vi "Audio_Transformation_Setted_Frequency_v008.vi"() -> ()   [LabVIEW 2019]
uses:
  <vilib>/sound2/lvsound2.llb/Sound Data Format.ctl
  <vilib>/sound2/lvsound2.llb/Sound Input Read (DBL).vi
  <vilib>/addons/Time Frequency Analysis/Transform.llb/TFA Online Gabor Transform (Real).vi
  <vilib>/addons/_Advanced Signal Processing/NI_AdvSigProcTFA.lvlib
panel:
  out "u(t)":T1(graph)
  out "V(t)":T1(graph)
  out "Noise Speech":dbl[](graph)
  in  "Address selector":i32[](array[numeric])
  in  "Neuron Type":T2(ring)=enum."Phasic Spiking (PS)"
  out "max index(es)":i32
  out "max value":dbl
  out "Waveform Graph":dbl[](graph)
  out "Magnitude of Gabor Coefficients":dbl[][](graph)
  in  "Stop":bool
  # "Step two : Graph of the amplitude of the Gabor coefficient of the different bins"
  # "Step three : Spike Response of the neurons"
  # "Step one: Sound recorded from the computer"
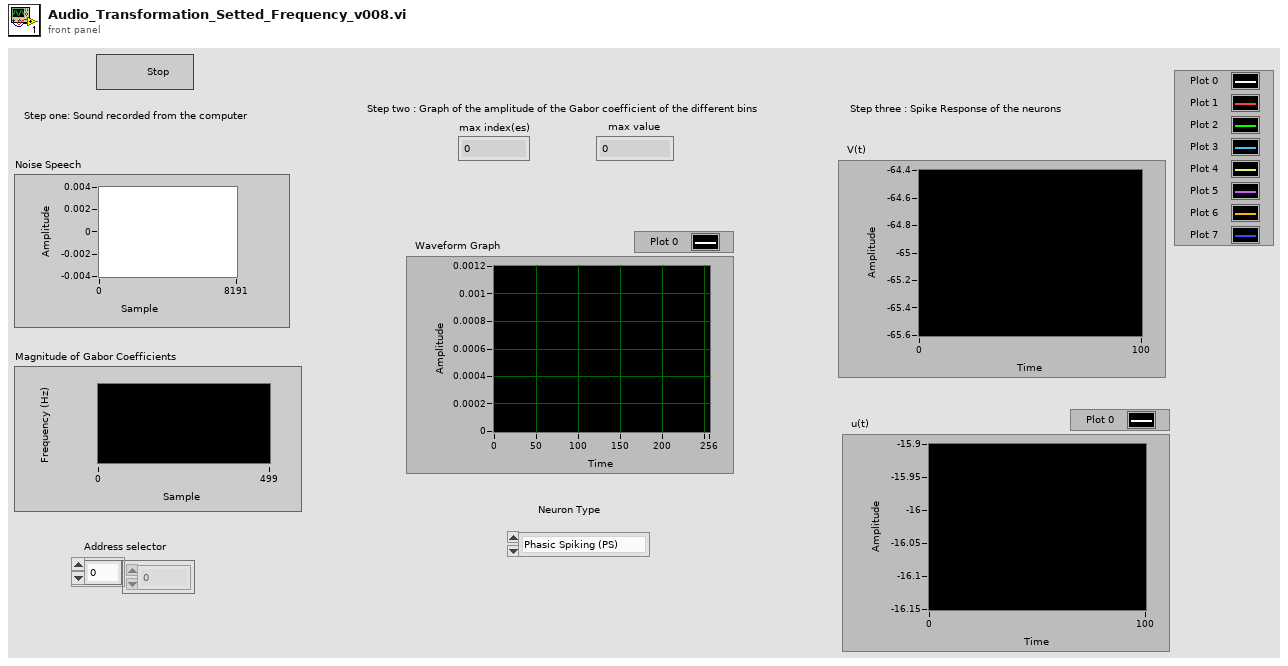
[diagram p1: front panel]
types:
  T1 = cluster{"[0]":dbl, "[1]":dbl, "[2]":dbl, "[3]":dbl, "[4]":dbl, "[5]":dbl, "[6]":dbl, "[7]":dbl}
  T2 = enum16{"Regular Spiking (RS)", "Intrinsically Bursting (IB)", "Chattering (CH)", "Fast Spiking (FS)", "Thalamo-Cortical 1 (TC1)", "Thalamo-Cortical 2 (TC2)", "Resonator (RZ)", "Low-Threshold Spiking (LTS)", "Phasic Spiking (PS)"}
  T3 = typedef "Sound Data Format.ctl" = cluster{"sample rate (S/s)":dbl, "number of channels":i32, "bits per sample":i32}
  T4 = cluster{"analysis window":dbl[], "dM (time steps)":i32, "N (frequency bins)":i32}
  T5 = typedef "Sound Input Task ID.ctl" = u32
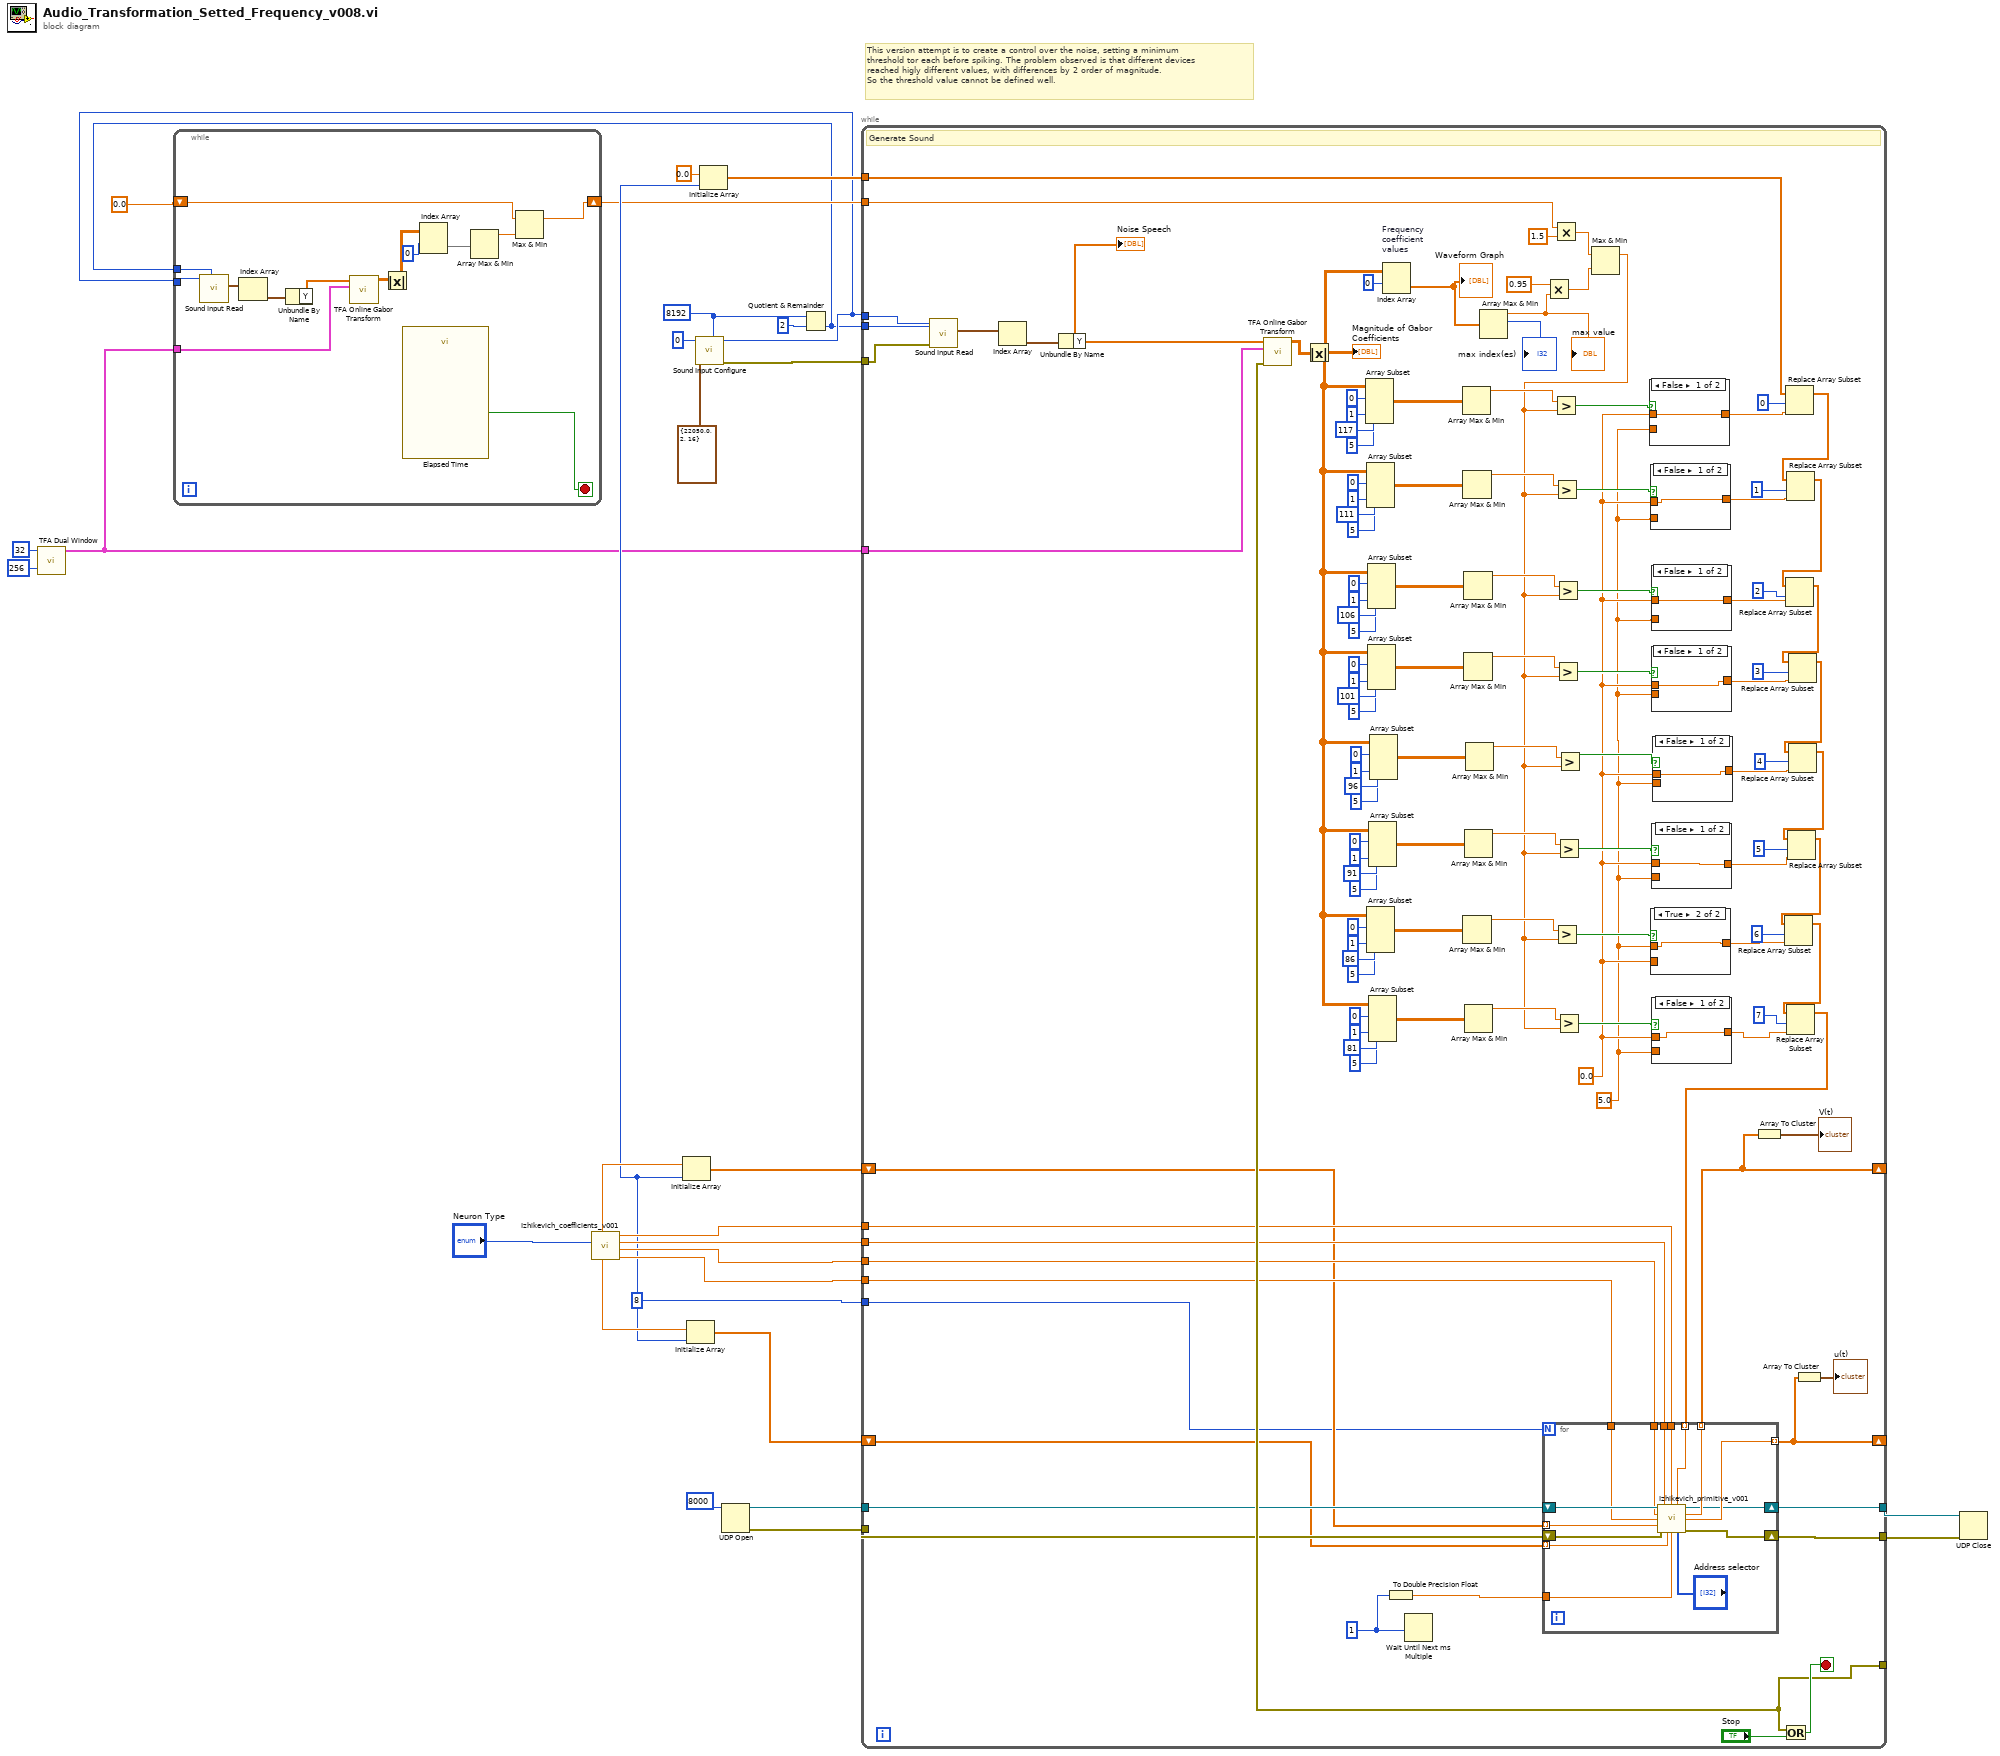
[diagram p0: block diagram]
diagram:
  w8 = 8
  w15 = 8192 ("number of samples/ch")
  # "This version attempt is to create a control over the noise, setting a minimum\nthreshold tor each before spiking. The problem observed is that different devices\nreached higly different values, with differences by 2 order of magnitude.\nSo the threshold value cannot be defined well."
  n1 = call <vilib>:"TFA Dual Window.vi"("N (frequency bins)"=256, "dM (time steps)"=32) -> ("analysis info"=w5:T4)  [unwired: 7 in, 2 out]
  n2 = call "Izhikevich_coefficients_v001.vi"("Neuron Type"="Neuron Type") -> ("d"=w23:dbl, "c"=w24:dbl, "b"=w25:dbl, "a"=w26:dbl, "u0"=w10:dbl, "v0"=w12:dbl)  [unwired: 3 in]
  n3 = Initialize Array(w12, w8) -> (w11:dbl[])
  n4 = Initialize Array(w10, w8) -> (w9:dbl[])
  n5 = call <vilib>:"Sound Input Configure.vi"("number of samples/ch"=w15, "sound format"=T3 {"sample rate (S/s)"=22050.0, "number of channels"=2, "bits per sample"=16}, "device ID"=u32 0) -> ("error out"=w13:errorcluster, "task ID"=w2:T5)  [unwired: 7 in]
  n6 = Initialize Array(0.0 ("element"), w8) -> (w6:dbl[])
  n7 = UDP Open(11:u16 8000 ("port")) -> (port=w21:refnum<k16>, 0:w20:errorcluster)  [unwired: 4 in, 1 out]
  n8 = Quotient & Remainder(x=w15, y=2) -> (floor(x/y)=w1:i32)  [unwired: 1 out]
  n9 = while {
    tunnel: w5 -> [w41]
    shift-right: [w33] -> w3
    shift-left: 0.0 -> [w34]
    tunnel: w2 -> [w31]
    tunnel: w1 -> [w30]
    stop <- w32 stop-if-true
    n10 = call-poly <vilib>:"Sound Input Read.vi"("number of samples/ch"=w30, "task ID"=w31) -> ("data"=w42:waveform(dbl)[])  [unwired: 7 in, 2 out]
    n11 = Index Array(array=w42) -> (element=w43:waveform(dbl))  [unwired: 1 in]
    n12 = Unbundle By Name(w43) -> ("Y"=w40:dbl[])
    n13 = call-poly <vilib>:"TFA Online Gabor Transform.vi"("transform info"=w41, "signal"=w40) -> ("Gabor coef"=w39:cdb[][])  [unwired: 7 in, 2 out]
    n14 = Absolute Value(x=w39) -> (abs(x)=w37:dbl[][])
    n15 = call "Elapsed Time"() -> ("Time has Elapsed"=w32:bool)  [unwired: 12 in, 7 out]
    n16 = Index Array(array=w37, index (row)=0) -> (element=w36:dbl[])  [unwired: 1 in]
    n17 = Array Max & Min(array=w36) -> (max value=w35:dbl)  [unwired: 3 out]
    n18 = Max & Min(x=w34, y=w35) -> (max(x,y)=w33:dbl)  [unwired: 1 out]
  }
  n19 = while {
    tunnel: [w158] -> _
    tunnel: w5 -> [w163]
    shift-right: [w57] -> _
    shift-left: w11 -> [w147]
    shift-right: [w55] -> _
    shift-left: w9 -> [w146]
    tunnel: w26 -> [w157]
    tunnel: w25 -> [w156]
    tunnel: w24 -> [w154]
    tunnel: w23 -> [w153]
    tunnel: w21 -> [w155]
    tunnel: w20 -> [w152]
    tunnel: [w149] -> w19
    tunnel: [w148] -> w18
    tunnel: w2 -> [w144]
    tunnel: w13 -> [w143]
    tunnel: w1 -> [w145]
    tunnel: w8 -> [w139]
    tunnel: w6 -> [w111]
    tunnel: w3 -> [w51]
    stop <- w164 stop-if-true
    w45 = 5.0
    w46 = 0.0
    w151 = u32 1 ("millisecond multiple")
    # "Generate Sound"
    n20 = call-poly <vilib>:"Sound Input Read.vi"("number of samples/ch"=w145, "error in (no error)"=w143, "task ID"=w144) -> ("data"=w141:waveform(dbl)[])  [unwired: 6 in, 2 out]
    n21 = Index Array(array=w141) -> (element=w142:waveform(dbl))  [unwired: 1 in]
    n22 = Unbundle By Name(w142) -> ("Y"=w140:dbl[])
    "Noise Speech" <- w140
    n23 = call-poly <vilib>:"TFA Online Gabor Transform.vi"("transform info"=w163, "signal"=w140) -> ("error out"=w158:errorcluster, "Gabor coef"=w162:cdb[][])  [unwired: 7 in, 1 out]
    n24 = Absolute Value(x=w162) -> (abs(x)=w60:dbl[][])
    "Magnitude of Gabor Coefficients" <- w60
    n25 = Array Subset(array=w60, index (row)=0 ("index"), length (row)=1 ("length"), index (col)=117 ("index"), length (col)=5 ("length")) -> (w134:dbl[][])
    n26 = Array Subset(array=w60, index (row)=0 ("index"), length (row)=1 ("length"), index (col)=111 ("index"), length (col)=5 ("length")) -> (w127:dbl[][])
    n27 = Array Subset(array=w60, index (row)=0 ("index"), length (row)=1 ("length"), index (col)=86 ("index"), length (col)=5 ("length")) -> (w74:dbl[][])
    n28 = Array Subset(array=w60, index (row)=0 ("index"), length (row)=1 ("length"), index (col)=106 ("index"), length (col)=5 ("length")) -> (w116:dbl[][])
    n29 = Array Subset(array=w60, index (row)=0 ("index"), length (row)=1 ("length"), index (col)=101 ("index"), length (col)=5 ("length")) -> (w104:dbl[][])
    n30 = Array Subset(array=w60, index (row)=0 ("index"), length (row)=1 ("length"), index (col)=91 ("index"), length (col)=5 ("length")) -> (w84:dbl[][])
    n31 = Array Subset(array=w60, index (row)=0 ("index"), length (row)=1 ("length"), index (col)=81 ("index"), length (col)=5 ("length")) -> (w64:dbl[][])
    n32 = Array Subset(array=w60, index (row)=0 ("index"), length (row)=1 ("length"), index (col)=96 ("index"), length (col)=5 ("length")) -> (w94:dbl[][])
    n33 = Index Array "Frequency \ncoefficient \nvalues"(array=w60, index (row)=0) -> (element=w160:dbl[])  [unwired: 1 in]
    "Waveform Graph" <- w160
    n34 = To Double Precision Float(number=w151) -> (double precision float=w150:dbl)
    n35 = Wait Until Next ms Multiple(millisecond multiple=w151) -> ()  [unwired: 1 out]
    n36 = Array Max & Min(array=w134) -> (max value=w133:dbl)  [unwired: 3 out]
    n37 = Array Max & Min(array=w127) -> (max value=w126:dbl)  [unwired: 3 out]
    n38 = Array Max & Min(array=w74) -> (max value=w73:dbl)  [unwired: 3 out]
    n39 = Array Max & Min(array=w116) -> (max value=w115:dbl)  [unwired: 3 out]
    n40 = Array Max & Min(array=w104) -> (max value=w103:dbl)  [unwired: 3 out]
    n41 = Array Max & Min(array=w84) -> (max value=w83:dbl)  [unwired: 3 out]
    n42 = Array Max & Min(array=w64) -> (max value=w63:dbl)  [unwired: 3 out]
    n43 = Array Max & Min(array=w94) -> (max value=w93:dbl)  [unwired: 3 out]
    n44 = Array Max & Min(array=w160) -> (max value=w48:dbl, max index (indices)=→"max index(es)":i32)  [unwired: 2 out]
    "max value" <- w48
    n45 = Multiply(x=0.95 ("y"), y=w48) -> (x*y=w49:dbl)
    n46 = Multiply(x=w51, y=1.5) -> (x*y=w50:dbl)
    n47 = Max & Min(x=w50, y=w49) -> (max(x,y)=w53:dbl)  [unwired: 1 out]
    n48 = Greater?(x=w133, y=w53) -> (0:w132:bool)
    n49 = Greater?(x=w126, y=w53) -> (0:w125:bool)
    n50 = Greater?(x=w73, y=w53) -> (0:w72:bool)
    n51 = Greater?(x=w115, y=w53) -> (0:w114:bool)
    n52 = Greater?(x=w103, y=w53) -> (0:w102:bool)
    n53 = Greater?(x=w83, y=w53) -> (0:w82:bool)
    n54 = Greater?(x=w63, y=w53) -> (0:w62:bool)
    n55 = Greater?(x=w93, y=w53) -> (0:w92:bool)
    n56 = case shown="False" w132 {
      tunnel: [w180 w181] -> w124
      tunnel: w46 -> [w180 _]
      tunnel: w45 -> [_ w181]
      frame False {
      }
      frame True {
      }
    }
    n57 = case shown="False" w125 {
      tunnel: [w178 w179] -> w121
      tunnel: w46 -> [w178 _]
      tunnel: w45 -> [_ w179]
      frame False {
      }
      frame True {
      }
    }
    n58 = case shown="True" w72 {
      tunnel: [w168 w169] -> w70
      tunnel: w46 -> [w168 _]
      tunnel: w45 -> [_ w169]
      frame False {
      }
      frame True {
      }
    }
    n59 = case shown="False" w114 {
      tunnel: [w176 w177] -> w112
      tunnel: w46 -> [w176 _]
      tunnel: w45 -> [_ w177]
      frame False {
      }
      frame True {
      }
    }
    n60 = case shown="False" w102 {
      tunnel: [w174 w175] -> w100
      tunnel: w46 -> [w174 _]
      tunnel: w45 -> [_ w175]
      frame False {
      }
      frame True {
      }
    }
    n61 = case shown="False" w82 {
      tunnel: [w170 w171] -> w80
      tunnel: w46 -> [w170 _]
      tunnel: w45 -> [_ w171]
      frame False {
      }
      frame True {
      }
    }
    n62 = case shown="False" w62 {
      tunnel: [w166 w167] -> w44
      tunnel: w46 -> [w166 _]
      tunnel: w45 -> [_ w167]
      frame False {
      }
      frame True {
      }
    }
    n63 = case shown="False" w92 {
      tunnel: [w172 w173] -> w90
      tunnel: w46 -> [w172 _]
      tunnel: w45 -> [_ w173]
      frame False {
      }
      frame True {
      }
    }
    n64 = Or(x=w158, y="Stop") -> (x .or. y?=w164:bool)
    n65 = Replace Array Subset(array=w111, new element=w124, index=0) -> (w110:dbl[])
    n66 = Replace Array Subset(array=w110, new element=w121, index=1) -> (w109:dbl[])
    n67 = Replace Array Subset(array=w109, new element=w112, index=2) -> (w99:dbl[])
    n68 = Replace Array Subset(array=w99, new element=w100, index=3) -> (w89:dbl[])
    n69 = Replace Array Subset(array=w89, new element=w90, index=4) -> (w79:dbl[])
    n70 = Replace Array Subset(array=w79, new element=w80, index=5) -> (w69:dbl[])
    n71 = Replace Array Subset(array=w69, new element=w70, index=6) -> (w59:dbl[])
    n72 = Replace Array Subset(array=w59, new element=w44, index=7) -> (w58:dbl[])
    n73 = for {
      N: w139 -> [_]
      tunnel: w157 -> [w196]
      tunnel: w156 -> [w195]
      tunnel: w154 -> [w193]
      tunnel: w153 -> [w192]
      tunnel: w150 -> [w189]
      tunnel: [w188] -> w57 mode=indexing
      tunnel: [w187] -> w55 mode=indexing
      tunnel: w147 -> [w184] mode=indexing
      tunnel: w146 -> [w183] mode=indexing
      shift-right: [w185] -> w148
      shift-left: w155 -> [w194]
      shift-right: [w186] -> w149
      shift-left: w152 -> [w191]
      tunnel: w58 -> [w182] mode=indexing
      n74 = call "Izhikevich_primitive_v001.vi"("UDP Network Connection in"=w194, "b"=w195, "a"=w196, "I"=w182, "c"=w193, "d"=w192, "v(t)"=w184, "error in (no error)"=w191, "u(t)"=w183, "Numeric"=w189, "Address selector"="Address selector") -> ("UDP Network Connection out"=w185:refnum<k16>, "v(t+dt)"=w188:dbl, "u(t+dt)"=w187:dbl, "error out"=w186:errorcluster)  [unwired: 1 in]
    }
    n75 = Array To Cluster(array=w57) -> (cluster=→"V(t)":T1)
    n76 = Array To Cluster(array=w55) -> (cluster=→"u(t)":T1)
  }
  n77 = UDP Close(connection ID=w18, 8:w19) -> ()  [unwired: 2 out]
